vi "Change Channel.vi"(7 "Channel Index":i32, 8 "error in (no error)":errorcluster, 10 "SD Control Refs in":T1, 11 "SD Module in":refnum<class "SD Module.lvclass">) -> (0 "error out":errorcluster, 2 "SD Control Refs out":T1, 3 "SD Module out":refnum<class "SD Module.lvclass">)   [LabVIEW 2017, in "Modules.lvlib" / "SD Module.lvclass"]
uses:
  SD Module.lvclass
  Type Defs/SD Control Refs.ctl
  Type Defs/Main Control Refs.ctl
  Type Defs/Counter Control Refs.ctl
  Type Defs/CDO Control Refs.ctl
  Type Defs/PWM Control Refs.ctl
  Type Defs/Quadrature Control Refs.ctl
  SD Module.lvclass/SD Module.ctl
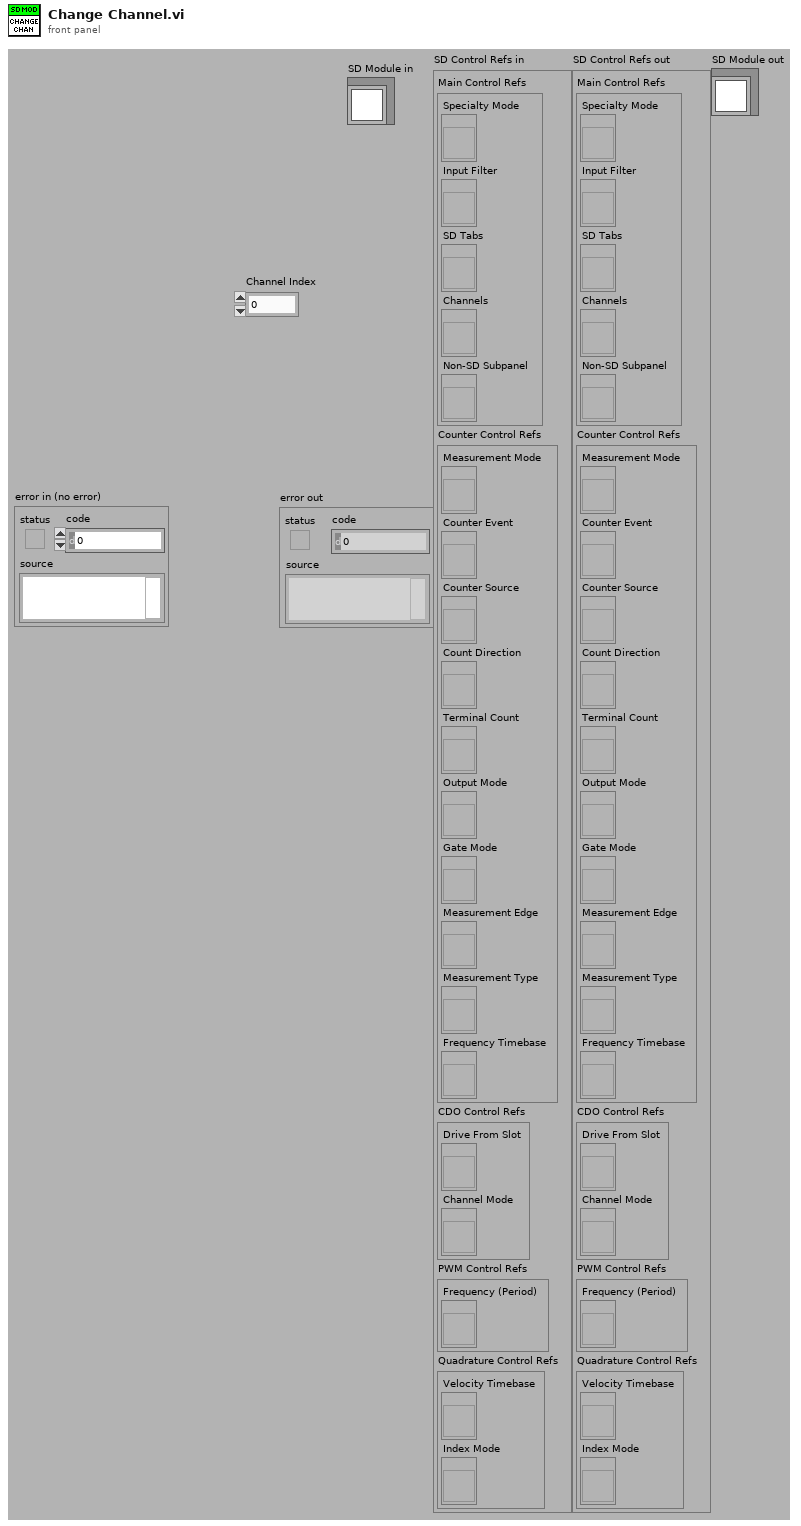
[diagram p1: front panel]
types:
  T1 = typedef "Modules.lvlib/SD Module.lvclass/SD Control Refs.ctl" = cluster{"Main Control Refs":T2, "Counter Control Refs":T3, "CDO Control Refs":T4, "PWM Control Refs":T5, "Quadrature Control Refs":T6}
  T2 = typedef "Modules.lvlib/SD Module.lvclass/Main Control Refs.ctl" = cluster{"Specialty Mode":refnum<vi>, "Input Filter":refnum<vi>, "SD Tabs":refnum<vi>, "Channels":refnum<vi>, "Non-SD Subpanel":refnum<vi>}
  T3 = typedef "Modules.lvlib/SD Module.lvclass/Counter Control Refs.ctl" = cluster{"Measurement Mode":refnum<vi>, "Counter Event":refnum<vi>, "Counter Source":refnum<vi>, "Count Direction":refnum<vi>, "Terminal Count":refnum<vi>, "Output Mode":refnum<vi>, "Gate Mode":refnum<vi>, "Measurement Edge":refnum<vi>, "Measurement Type":refnum<vi>, "Frequency Timebase":refnum<vi>}
  T4 = typedef "Modules.lvlib/SD Module.lvclass/CDO Control Refs.ctl" = cluster{"Drive From Slot":refnum<vi>, "Channel Mode":refnum<vi>}
  T5 = typedef "Modules.lvlib/SD Module.lvclass/PWM Control Refs.ctl" = cluster{"Frequency (Period)":refnum<vi>}
  T6 = typedef "Modules.lvlib/SD Module.lvclass/Quadrature Control Refs.ctl" = cluster{"Velocity Timebase":refnum<vi>, "Index Mode":refnum<vi>}
  T7 = typedef "Modules.lvlib/SD Module.lvclass/Counter Channel.ctl" = cluster{"Measurement Mode":u32, "Count Edges":T8, "Period Measurement":T9, "Pulse Width Measurement":T10, "Frequency Measurement":T11}
  T8 = typedef "Modules.lvlib/SD Module.lvclass/Count Edges.ctl" = cluster{"Counter Event":u32, "Counter Source":u32, "Counter Direction":u32, "Terminal Count":u32, "Output Mode":u32, "Gate Mode":u32}
  T9 = typedef "Modules.lvlib/SD Module.lvclass/Period Measurement.ctl" = cluster{"Measurement Edge":u32}
  T10 = typedef "Modules.lvlib/SD Module.lvclass/Pulse Width Measurement.ctl" = cluster{"Measurement Type":u32}
  T11 = typedef "Modules.lvlib/SD Module.lvclass/Frequency Measurement.ctl" = cluster{"Measurement Edge":u32, "Measurement Timebase":u32}
  T12 = typedef "Modules.lvlib/SD Module.lvclass/CDO Channel.ctl" = cluster{"Counter driven enabled":bool}
  T13 = typedef "Modules.lvlib/SD Module.lvclass/PWM Channel.ctl" = cluster{"PWM frequency":u32}
  T14 = typedef "Modules.lvlib/SD Module.lvclass/Quadrature Channel.ctl" = cluster{"Timebase":u32, "Index Mode":u32}
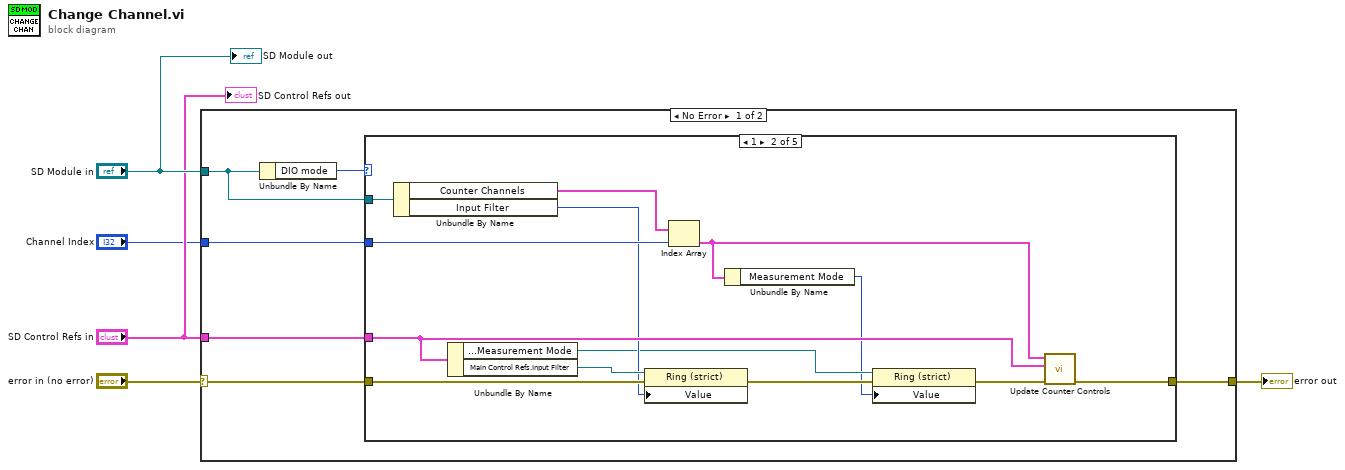
[diagram p0: block diagram]
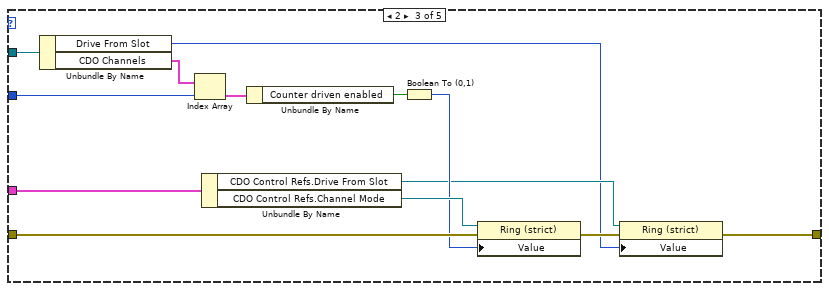
[diagram p3: hidden frame]
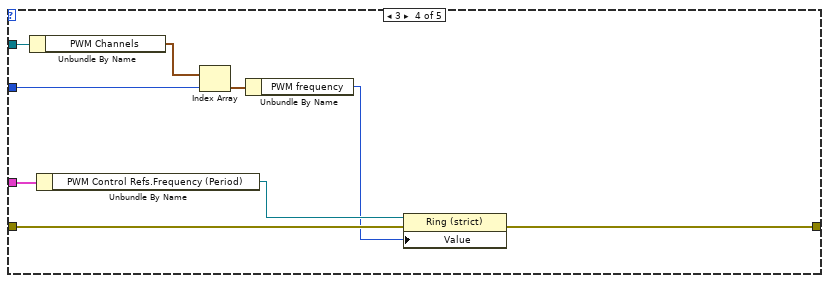
[diagram p4: hidden frame]
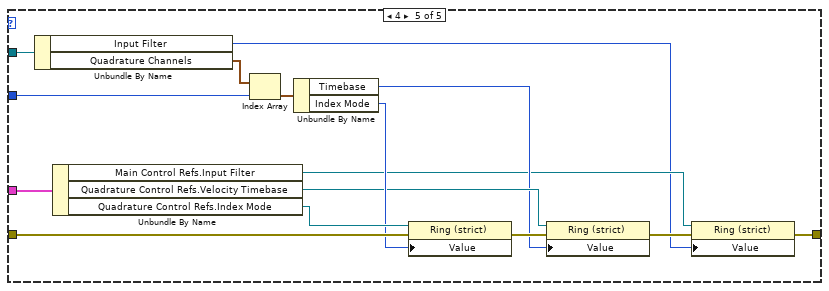
[diagram p5: hidden frame]
diagram:
  n1 = case shown="No Error" "error in (no error)" {
    selector: "error in (no error)" -> [w7 w63]
    tunnel: [w6 w63] -> w3
    tunnel: "SD Control Refs in" -> [w9 _]
    tunnel: "SD Module in" -> [w10 _]
    tunnel: "Channel Index" -> [w8 _]
    frame No Error {
      n2 = Unbundle By Name(w10) -> ("DIO mode"=w11:u32)
      n3 = case shown="1" w11 {
        tunnel: w10 -> [_ w24 w38 w47 w62]
        tunnel: w9 -> [_ w20 w34 w43 w58]
        tunnel: w8 -> [_ w23 w36 w45 w60]
        tunnel: w7 -> [w12 w22 w33 w42 w57]
        tunnel: [w12 w21 w26 w39 w48] -> w6
        frame 0, Default {
        }
        frame 1 {
          n4 = Unbundle By Name(w24) -> ("Counter Channels"=w25:T7[], "Input Filter"=w18:u32)
          n5 = Unbundle By Name(w20) -> ("Counter Control Refs.Measurement Mode"=w16:refnum<vi>, "Main Control Refs.Input Filter"=w19:refnum<vi>)
          n6 = property class="Ring (strict)"(reference=w19, error in=w22, "Value"=w18) -> (error out=w17:errorcluster)  [unwired: 1 out]
          n7 = Index Array(array=w25, index=w23) -> (element=w15:T7)
          n8 = Unbundle By Name(w15) -> ("Measurement Mode"=w14:u32)
          n9 = property class="Ring (strict)"(reference=w16, error in=w17, "Value"=w14) -> (error out=w13:errorcluster)  [unwired: 1 out]
          n10 = call "Update Counter Controls.vi"("error in (no error)"=w13, "SD Control Refs in"=w20, "Counter Channel"=w15) -> ("error out"=w21:errorcluster)  [unwired: 8 in]
        }
        frame 2 {
          n11 = Unbundle By Name(w38) -> ("Drive From Slot"=w27:u32, "CDO Channels"=w37:T12[])
          n12 = Index Array(array=w37, index=w36) -> (element=w35:T12)
          n13 = Unbundle By Name(w34) -> ("CDO Control Refs.Drive From Slot"=w28:refnum<vi>, "CDO Control Refs.Channel Mode"=w31:refnum<vi>)
          n14 = Unbundle By Name(w35) -> ("Counter driven enabled"=w32:bool)
          n15 = Boolean To (0,1)(Boolean=w32) -> (0, 1=w30:i16)
          n16 = property class="Ring (strict)"(reference=w31, error in=w33, "Value"=w30) -> (error out=w29:errorcluster)  [unwired: 1 out]
          n17 = property class="Ring (strict)"(reference=w28, error in=w29, "Value"=w27) -> (error out=w26:errorcluster)  [unwired: 1 out]
        }
        frame 3 {
          n18 = Unbundle By Name(w47) -> ("PWM Channels"=w46:T13[])
          n19 = Unbundle By Name(w43) -> ("PWM Control Refs.Frequency (Period)"=w41:refnum<vi>)
          n20 = Index Array(array=w46, index=w45) -> (element=w44:T13)
          n21 = Unbundle By Name(w44) -> ("PWM frequency"=w40:u32)
          n22 = property class="Ring (strict)"(reference=w41, error in=w42, "Value"=w40) -> (error out=w39:errorcluster)  [unwired: 1 out]
        }
        frame 4 {
          n23 = Unbundle By Name(w62) -> ("Input Filter"=w49:u32, "Quadrature Channels"=w61:T14[])
          n24 = Unbundle By Name(w58) -> ("Main Control Refs.Input Filter"=w51:refnum<vi>, "Quadrature Control Refs.Velocity Timebase"=w53:refnum<vi>, "Quadrature Control Refs.Index Mode"=w56:refnum<vi>)
          n25 = Index Array(array=w61, index=w60) -> (element=w59:T14)
          n26 = Unbundle By Name(w59) -> ("Timebase"=w52:u32, "Index Mode"=w55:u32)
          n27 = property class="Ring (strict)"(reference=w56, error in=w57, "Value"=w55) -> (error out=w54:errorcluster)  [unwired: 1 out]
          n28 = property class="Ring (strict)"(reference=w53, error in=w54, "Value"=w52) -> (error out=w50:errorcluster)  [unwired: 1 out]
          n29 = property class="Ring (strict)"(reference=w51, error in=w50, "Value"=w49) -> (error out=w48:errorcluster)  [unwired: 1 out]
        }
      }
    }
    frame Error {
    }
  }
  "error out" <- w3
  "SD Control Refs out" <- "SD Control Refs in"
  "SD Module out" <- "SD Module in"
